vi "Clean.vi"(0 "NIPKG_LV in":refnum<class "NIPKG_LV.lvclass">) -> (4 "NIPKG_LV out":refnum<class "NIPKG_LV.lvclass">)   [LabVIEW 2017, in "CL_G3_VIComponentBuilder.lvlib" / "NIPKG_LV.lvclass"]
doc: "Unregisters the NI Package found in the Component's export directory form the build machine feed and deletes the NI Package."
uses:
  NIPKG_LV.lvclass
  C:/Tool Chain Support/Software Module Builder/Source/Exports/Exports/Export.lvclass
  Exports/Export.lvclass/Export.ctl
  NIPKG_LV.lvclass/NIPKG_LV.ctl
  Exports/Accessors/Write Built Export's Full Path.vi
  Exports/Accessors/Read Component Export Dir.vi
  Exports/Accessors/Read unique Name.vi
  Accessors/Read Build Machine Feed Folderpath.vi
  Exports/Accessors/Write Export Operation Errors.vi
  Exports/Accessors/Read Export Operation Errors.vi
  <vilib>/Utility/file.llb/Is Path and Not Empty.vi
  NI Build Specification_LV/NI Build Specification_LV.lvclass
  <userlib>/_Cirrus Logic/NI Package Manager API/Source/TCS_NIPKG_API.lvlib
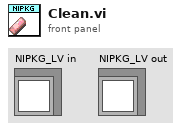
[diagram p1: front panel]
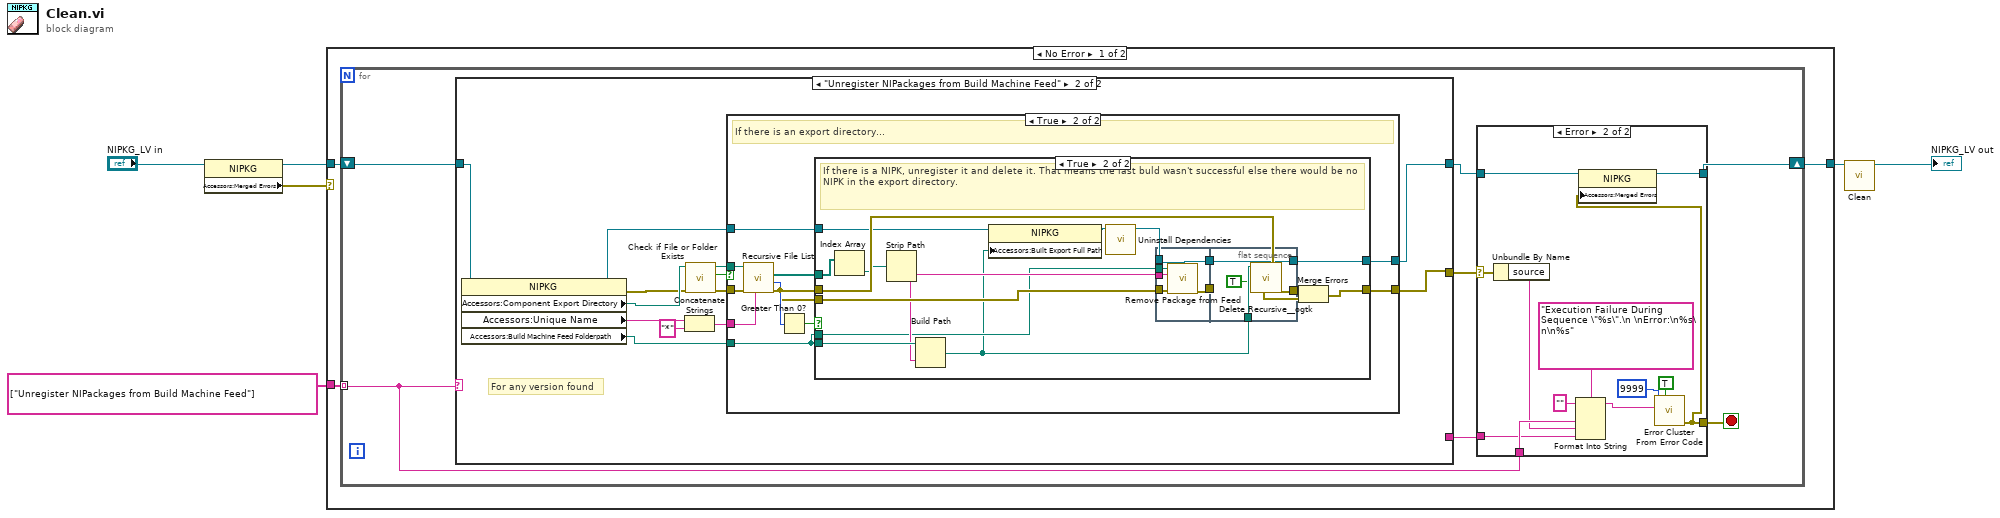
[diagram p0: block diagram]
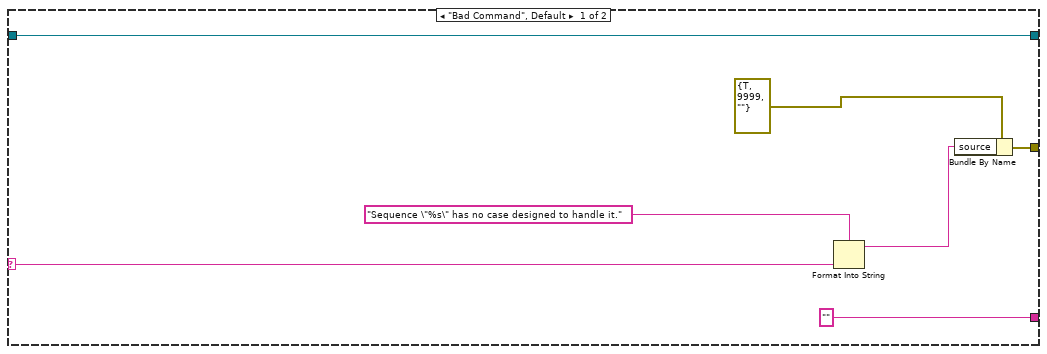
[diagram p2: hidden frame]
diagram:
  n1 = property class="NIPKG"(reference="NIPKG_LV in") -> (reference out=w4:refnum<class "NIPKG_LV.lvclass">, "Accessors:Merged Errors"=w6:errorcluster)  [unwired: 1 in, 1 out]
  n2 = case shown="No Error" w6 {
    tunnel: string[] ["Unregister NIPackages from Build Machine Feed"] ("Sequences") -> [w9 _]
    tunnel: w4 -> [w8 w91]
    tunnel: [w7 w91] -> w2
    frame No Error {
      n3 = for {
        tunnel: w9 -> [w14] mode=indexing
        shift-right: [w10] -> w7
        shift-left: w8 -> [w16]
        stop <- w12 stop-if-true
        n4 = case shown="\"Unregister NIPackages from Build Machine Feed\"" w14 {
          selector: w14 -> [w18 _]
          tunnel: w16 -> [w23 w28]
          tunnel: [w23 w24] -> w11
          tunnel: [w20 w27] -> w15
          tunnel: ["" ("Accessors:Name") _] -> w13
          frame "Bad Command", Default {
            n5 = Format Into String(format string="Sequence \"%s\" has no case designed to handle it.", w18) -> (resulting string=w17:string)  [unwired: 2 in, 1 out]
            n6 = Bundle By Name(cluster=errorcluster {"status"=TRUE, "code"=9999, "source"=""} ("error out"), "source"=w17) -> (w20:errorcluster)
          }
          frame "Unregister NIPackages from Build Machine Feed" {
            # "For any version found"
            n7 = property class="NIPKG"(reference=w28) -> (reference out=w25:refnum<class "NIPKG_LV.lvclass">, error out=w32:errorcluster, "Accessors:Component Export Directory"=w36:path, "Accessors:Unique Name"=w34:string, "Accessors:Build Machine Feed Folderpath"=w26:path)  [unwired: 1 in]
            n8 = Concatenate Strings(w34, "*" ("string")) -> (w35:string)
            n9 = call <vilib>:"Check if File or Folder Exists.vi"("error in (no error)"=w32, "path"=w36) -> ("error out"=w33:errorcluster, "file or folder exists?"=w31:bool, "dup path"=w30:path)  [unwired: 7 in]
            n10 = case shown="True" w31 {
              tunnel: w35 -> [_ w49]
              tunnel: w30 -> [_ w45]
              tunnel: w33 -> [w38 w44]
              tunnel: [w38 w43] -> w27
              tunnel: w26 -> [_ w40]
              tunnel: w25 -> [w37 w42]
              tunnel: [w37 w39] -> w24
              frame False {
              }
              frame True {
                # "If there is an export directory..."
                n11 = call <vilib>:"Recursive File List.vi"("pattern"=w49, "error in (no error)"=w44, "Folder Path"=w45) -> ("error out"=w41:errorcluster, "Number of Files"=w48:i32, "All Files in Dir"=w47:path[])  [unwired: 4 in, 2 out]
                n12 = Greater Than 0?(x=w48) -> (x > 0?=w46:bool)
                n13 = case shown="True" w46 {
                  tunnel: w47 -> [_ w67]
                  tunnel: w41 -> [w51 w66]
                  tunnel: [w51 w65] -> w43
                  tunnel: w40 -> [_ w60]
                  tunnel: w42 -> [w50 w62]
                  tunnel: w41 -> [_ w58]
                  tunnel: w40 -> [_ w56]
                  tunnel: [w50 w53] -> w39
                  frame False {
                  }
                  frame True {
                    # "If there is a NIPK, unregister it and delete it. That means the last buld wasn't successful else there would be no NIPK in the export directory."
                    n14 = Index Array(array=w67) -> (element=w64:path)  [unwired: 1 in]
                    n15 = Strip Path(path=w64) -> (name=w57:string)  [unwired: 1 out]
                    n16 = Build Path(base path=w60, name or relative path=w57) -> (appended path=w52:path)
                    n17 = property class="NIPKG"(reference=w62, "Accessors:Built Export Full Path"=w52) -> (reference out=w61:refnum<class "NIPKG_LV.lvclass">)  [unwired: 1 in, 1 out]
                    n18 = call-dynamic "Uninstall Dependencies.vi"("NIPKG_LV in"=w61) -> ("NIPKG_LV out"=w55:refnum<class "NIPKG_LV.lvclass">)  [unwired: 14 in]
                    n19 = flat-sequence {
                      tunnel: [w69] -> w59
                      tunnel: w58 -> [w72]
                      tunnel: w57 -> [w71]
                      tunnel: w56 -> [w70]
                      tunnel: w55 -> [w68]
                      tunnel: [w68] -> w54
                      tunnel: [w76] -> w63
                      tunnel: w52 -> [w75]
                      tunnel: w59 -> [_]
                      tunnel: [w73] -> w53
                      tunnel: w54 -> [w73]
                      frame #0 {
                        n20 = call <userlib>:"Remove Package from Feed.vi"("error in"=w72, "package filename"=w71, "feed folderpath"=w70) -> ("error out"=w69:errorcluster)  [unwired: 8 in]
                      }
                      frame #1 {
                        n21 = call <userlib>:"Delete Recursive__ogtk.vi"("Ignore Read-Only? (FALSE)"=TRUE, "Path"=w75) -> ("error out"=w76:errorcluster)  [unwired: 8 in, 1 out]
                      }
                    }
                    n22 = Merge Errors(w66, w63) -> (w65:errorcluster)
                  }
                }
              }
            }
          }
        }
        n23 = case shown="Error" w15 {
          selector: w15 -> [w78 w84]
          tunnel: [w78 w79] -> w12
          tunnel: w14 -> [_ w87]
          tunnel: w13 -> [_ w82]
          tunnel: w11 -> [w77 w81]
          tunnel: [w77 w80] -> w10
          frame No Error {
          }
          frame Error {
            n24 = Unbundle By Name(w84) -> ("source"=w83:string)
            n25 = Format Into String(format string="Execution Failure During Sequence \"%s\".\n \nError:\n%s\n\n%s" ("error message (\"\")"), initial string="", w87, w83, w82) -> (resulting string=w88:string)  [unwired: 1 in, 1 out]
            n26 = call <vilib>:"Error Cluster From Error Code.vi"("show call chain? (False)"=TRUE, "error message (\"\")"=w88, "error code (0)"=9999) -> ("error out"=w79:errorcluster)  [unwired: 6 in]
            n27 = property class="NIPKG"(reference=w81, "Accessors:Merged Errors"=w79) -> (reference out=w80:refnum<class "NIPKG_LV.lvclass">)  [unwired: 1 in, 1 out]
          }
        }
      }
    }
    frame Error {
    }
  }
  n28 = call-parent "Clean.vi"("NI Build Specification_LV in"=w2) -> ("NI Build Specification_LV out"=→"NIPKG_LV out":refnum<class "NIPKG_LV.lvclass">)  [unwired: 14 in]
